vi "Globals.vi"() -> ()   [LabVIEW 2018]
panel:
  in  "RESETs":dbl
  in  "SETs":dbl
  in  "READs":dbl
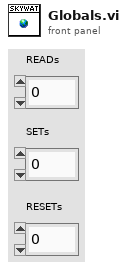
[diagram p1: front panel]
diagram:
